vi "exponential.ave.vi"(9 "continuous ave":i32, 10 "Array in":i32[](array[numeric]), 11 "CCD":i32[](array[numeric])) -> (3 "Array out":i32[](array[numeric]))   [LabVIEW 2022 SP3]
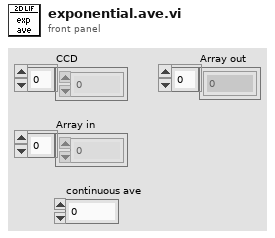
[diagram p1: front panel]
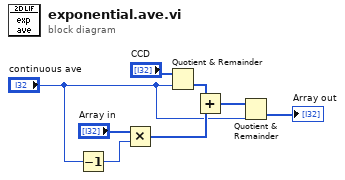
[diagram p0: block diagram]
diagram:
  n1 = Decrement(x="continuous ave") -> (x-1=w1:i32)
  n2 = Multiply(x="Array in", y=w1) -> (x*y=w7:i32[])
  n3 = Quotient & Remainder(x="CCD", y="continuous ave") -> (floor(x/y)=w6:i32[])  [unwired: 1 out]
  n4 = Add(x=w6, y=w7) -> (x+y=w5:i32[])
  n5 = Quotient & Remainder(x=w5, y="continuous ave") -> (floor(x/y)=→"Array out":i32[])  [unwired: 1 out]
